vi "FIU channel values to SPI 16bit SPI data.vi"(10 "FIU Channel values":dbl[](array[numeric])) -> (2 "data word":u16)   [LabVIEW 2014, in "SLSC configuration Shared.lvlib"]
uses:
  SLSC configuration Shared.lvlib
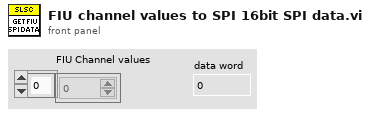
[diagram p1: front panel]
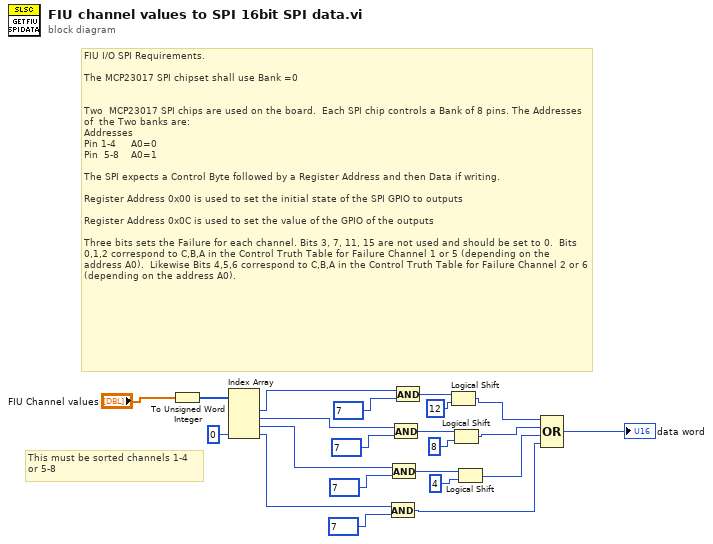
[diagram p0: block diagram]
diagram:
  # "This must be sorted channels 1-4\nor 5-8"
  # "FIU I/O SPI Requirements.\n\nThe MCP23017 SPI chipset shall use Bank =0 \n \n\nTwo  MCP23017 SPI chips are used on the board.  Each SPI chip controls a Bank of 8 pins. The Addresses of  the Two banks are:\nAddresses\nPin 1-4     A0=0\nPin  5-8    A0=1\n\nThe SPI expects a Control Byte followed by a Register Address and then Data if writing. \n\nRegister Address 0x00 is used to set the initial state of the SPI GPIO to outputs\n\nRegister Address 0x0C is used to set the value of the GPIO of the outputs\n\nThree bits sets the Failure for each channel. Bits 3, 7, 11, 15 are not used and should be set to 0.  Bits 0,1,2 correspond to C,B,A in the Control Truth Table for Failure Channel 1 or 5 (depending on the address A0).  Likewise Bits 4,5,6 correspond to C,B,A in the Control Truth Table for Failure Channel 2 or 6 (depending on the address A0)."
  n1 = To Unsigned Word Integer(number="FIU Channel values") -> (unsigned 16bit integer=w1:u16[])
  n2 = Index Array(array=w1, index #4=0 ("index")) -> (element #1=w5:u16, element #2=w9:u16, element #3=w10:u16, element #4=w11:u16)  [unwired: 3 in]
  n3 = And(x=w11, y=u16 7) -> (x .and. y?=w21:u16)
  n4 = And(x=w10, y=u16 7) -> (x .and. y?=w14:u16)
  n5 = And(x=w9, y=u16 7) -> (x .and. y?=w13:u16)
  n6 = And(x=w5, y=u16 7) -> (x .and. y?=w12:u16)
  n7 = Logical Shift(y=w12, x=u16 12) -> (x << y=w18:u16)
  n8 = Logical Shift(y=w13, x=u16 8) -> (x << y=w19:u16)
  n9 = Logical Shift(y=w14, x=u16 4) -> (x << y=w20:u16)
  n10 = Compound Arithmetic op=OR(w18, w19, w20, w21) -> (→"data word":u16)
